vi "Get Path.vi"(8 "error in (no error)":errorcluster, 11 "PropertyObjectFile in":refnum<class "PropertyObjectFile.lvclass">) -> (0 "error out":errorcluster, 2 "Path":path, 3 "PropertyObjectFile out":refnum<class "PropertyObjectFile.lvclass">)   [LabVIEW 2020, in "TSnax.lvlib" / "PropertyObjectFile.lvclass"]
uses:
  PropertyObjectFile.lvclass
  PropertyObjectFile.lvclass/PropertyObjectFile.ctl
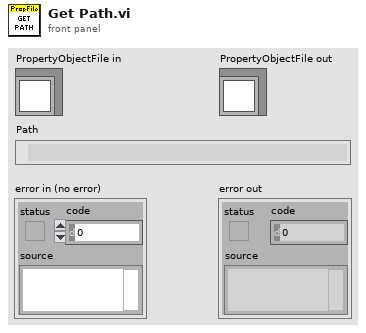
[diagram p1: front panel]
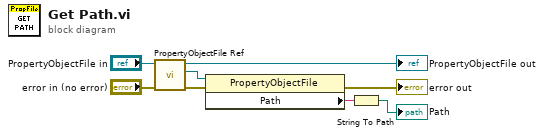
[diagram p0: block diagram]
diagram:
  n1 = call "PropertyObjectFile Ref.vi"("error in (no error)"="error in (no error)", "PropertyObjectFile in"="PropertyObjectFile in") -> ("error out"=w4:errorcluster, "PropertyObjectFile"=w5:refnum<k7>, "PropertyObjectFile out"=→"PropertyObjectFile out":refnum<class "PropertyObjectFile.lvclass">)  [unwired: 7 in]
  n2 = property class="PropertyObjectFile"(reference=w5, error in=w4) -> (error out=→"error out":errorcluster, "Path"=w2:string)  [unwired: 1 out]
  n3 = String To Path(string=w2) -> (path=→"Path":path)
